vi "NavbalLabVIEW(15-5-28.vi"() -> ()   [LabVIEW 2012] (continued)
            n1742 = Index Array(array=w713, index (col)=0 ("disabled index (col)")) -> (element=w715:string[])  [unwired: 1 in]
            n1743 = for {
              N: w706 -> [_]
              tunnel: w705 -> [w721] mode=indexing
              tunnel: w708 -> [w720] mode=indexing
              tunnel: [w719] -> w709 mode=indexing
              tunnel: w715 -> [w718] mode=indexing
              n1744 = Equal?(x=w718, y="W") -> (x = y?=w716:bool)
              n1745 = case shown="True" w716 {
                tunnel: w721 -> [w727 w735]
                tunnel: w720 -> [w724 w732]
                tunnel: [w722 w730] -> w719
                frame False {
                  n1746 = Decrement(x=w727) -> (x-1=w726:dbl)
                  n1747 = Divide(x=360.0, y=w724) -> (x/y=w723:dbl)
                  n1748 = Multiply(x=w723, y=w726) -> (x*y=w722:dbl)
                }
                frame True {
                  n1749 = Decrement(x=w735) -> (x-1=w734:dbl)
                  n1750 = Divide(x=360.0, y=w732) -> (x/y=w731:dbl)
                  n1751 = Multiply(x=w731, y=w734) -> (x*y=w729:dbl)
                  n1752 = Subtract(x=360.0, y=w729) -> (x-y=w730:dbl)
                }
              }
            }
            n1753 = Reshape Array(w709, 4 ("dimension size"), 1 ("dimension size")) -> (w712:dbl[][])
            n1754 = local write "Correction Phase"(w712) -> ()
          }
          frame #1 {
            w782 = i16 3 ("precision (6)")
            # "Add Correction \nto Baseline Vibes"
            # "Calc Effect of Masses"
            n1755 = local read "Startpt Complex"() -> (w743:cdb[][])
            n1756 = Divide(x="Correction Phase", y=180) -> (x/y=w807:T3)
            n1757 = Complex To Polar(r * e^(i*theta)=w743) -> (r=w795:dbl[][], theta=w796:dbl[][])
            n1758 = call-poly <vilib>:"Multiply.vi"("Real Scalar c"=3.141592653589793, "Real Matrix A"=w807) -> ("A * c"=w805:T3)
            n1759 = Divide(x=w796, y=3.141592653589793) -> (x/y=w792:dbl[][])
            n1760 = local read "Response Coefficients"() -> (w742:cdb[][])
            n1761 = call-poly <vilib>:"Polar To Complex.vi"("Argument Q"=w805, "Modulus r"="Correction Mag") -> ("Complex Matrix r*e^iQ"=w809:T15)
            n1762 = Multiply ("Multiply.vi")(x=w792, y=180) -> (x*y=w797:dbl[][])
            n1763 = call-poly <vilib>:"Matrix To Array.vi"("Real Matrix"=w795) -> ("Real 2D Array"=w770:dbl[][])
            n1764 = call-poly <vilib>:"Array To Matrix.vi"("Complex 2D Array"=w743) -> ("Complex Matrix"=w762:T15)
            n1765 = call-poly <vilib>:"A x B.vi"("B"=w809, "A"=w742) -> ("A x B"=w751:T15)  [unwired: 1 out]
            n1766 = Matrix Size(0:w797) -> (1:w799:i32)  [unwired: 1 out]
            n1767 = Index Array(array=w770, index (col)=0 ("disabled index (col)")) -> (element=w764:dbl[])  [unwired: 1 in]
            n1768 = call-poly <vilib>:"Add.vi"("Complex Matrix B"=w762, "Complex Matrix A"=w751) -> ("A + B"=w771:T15)
            n1769 = Matrix Size(0:w762) -> (1:w791:i32)  [unwired: 1 out]
            n1770 = Square(x=w764) -> (x^2=w768:dbl[])
            n1771 = for {
              N: w799 -> [_]
              tunnel: w797 -> [w813] mode=indexing
              tunnel: [w814] -> w798 mode=indexing
              n1772 = Index Array(array=w813, index=0) -> (element=w811:dbl)
              n1773 = Add(x=360.0, y=w811) -> (x+y=w815:dbl)
              n1774 = Less Than 0?(x=w811) -> (x < 0?=w816:bool)
              n1775 = Select(t=w815, s=w816, f=w811) -> (s? t:f=w814:dbl)
            }
            n1776 = Add Array Elements(numeric array=w768) -> (sum=w767:dbl)
            n1777 = call-poly <vilib>:"Complex To Polar.vi"("Complex Matrix r*e^iQ"=w771) -> ("Modulus r"=w737:T3, "Argument Q"=w757:T3)
            n1778 = Divide(x=w767, y=w791) -> (x/y=w766:dbl)
            n1779 = call-poly <vilib>:"Multiply.vi"("Real Scalar c"=180.0 ("y"), "Real Matrix A"=w757) -> ("A * c"=w759:T3)
            n1780 = Square Root(x=w766) -> (sqrt(x)=w765:dbl)
            n1781 = Divide(x=w759, y=3.141592653589793) -> (x/y=w761:T3)
            n1782 = Absolute Value(x=w765) -> (abs(x)=w778:dbl)
            n1783 = Round To Nearest(number=w761) -> (nearest integer value=w790:T3)
            n1784 = call-poly <vilib>:"Subtract.vi"("Real Matrix B"=w737, "Real Matrix A"=w795) -> ("A - B"=w773:T3)
            n1785 = call-poly <vilib>:"Matrix To Array.vi"("Real Matrix"=w737) -> ("Real 2D Array"=w752:dbl[][])
            n1786 = Matrix Size(0:w790) -> (1:w763:i32)  [unwired: 1 out]
            n1787 = Index Array(array=w752, index (col)=0 ("disabled index (col)")) -> (element=w772:dbl[])  [unwired: 1 in]
            n1788 = for {
              N: w763 -> [_]
              tunnel: w790 -> [w820] mode=indexing
              tunnel: [w821] -> w736 mode=indexing
              n1789 = Index Array(array=w820, index=0) -> (element=w818:dbl)
              n1790 = Add(x=360.0, y=w818) -> (x+y=w822:dbl)
              n1791 = Less Than 0?(x=w818) -> (x < 0?=w823:bool)
              n1792 = Select(t=w822, s=w823, f=w818) -> (s? t:f=w821:dbl)
            }
            "Predicted Phase" <- w736
            n1793 = Build Array (concatenate)(w795, w798, w737, w736, w773) -> (w774:T3)
            n1794 = Array Max & Min(array=w737) -> (max index (indices)=w750:i32[])  [unwired: 3 out]
            n1795 = Square(x=w772) -> (x^2=w754:dbl[])
            n1796 = Add Array Elements(numeric array=w754) -> (sum=w755:dbl)
            n1797 = Index Array(array=w750, index=0) -> (element=w748:i32)
            n1798 = Number To Fractional String(number=w774, precision (6)=w782) -> (F-format string=w775:string[][])  [unwired: 2 in]
            n1799 = Divide(x=w755, y=w791) -> (x/y=w756:dbl)
            n1800 = Number To Fractional String(number=w778, precision (6)=w782) -> (F-format string=w788:string)  [unwired: 2 in]
            n1801 = Square Root(x=w756) -> (sqrt(x)=w777:dbl)
            n1802 = Insert Into Array(array=w775, index (row)=w791, new element=string[] [] ("new element/subarray")) -> (w779:string[][])  [unwired: 1 in]
            n1803 = Bundle(w748, "disabled index (col)"=3) -> (w800:cluster{i32, "disabled index (col)":i32})  [unwired: 1 in]
            n1804 = Concatenate Strings("RMS: " ("string"), w788) -> (w789:string)
            n1805 = Replace Array Subset(array=w779, new element=w789, index (row)=w791, index (col)=0 ("disabled index (col)")) -> (w781:string[][])
            n1806 = property on="Prediction Results" class="MCListbox (strict)"("ActiveCell"=w800) -> (error out=w747:errorcluster)  [unwired: 2 in, 1 out]
            n1807 = Number To Fractional String(number=w777, precision (6)=w782) -> (F-format string=w784:string)  [unwired: 2 in]
            n1808 = Concatenate Strings("RMS: " ("string"), w784) -> (w786:string)
            n1809 = Replace Array Subset(array=w781, new element=w786, index (row)=w791, index (col)=2 ("disabled index (col)")) -> (w746:string[][])
            n1810 = property on="Prediction Results" class="MCListbox (strict)"(error in=w747, "CellBG"=u32 16759409) -> ()  [unwired: 1 in, 2 out]
            n1811 = call-poly <vilib>:"Matrix To Array.vi"("Real Matrix"=w737) -> ("Real 2D Array"=w740:dbl[][])
            n1812 = local read "Sensor Column"() -> (w741:string[])
            n1813 = Index Array(array=w740, index (col)=0 ("disabled index (col)")) -> (element=→"Predicted Mag":dbl[])  [unwired: 1 in]
            n1814 = Insert Into Array(array=w746, index (col)=0 ("disabled index (col)"), new element=w741) -> (w745:string[][])  [unwired: 1 in]
            n1815 = property on="Prediction Results" class="MCListbox (strict)"("ItemNames"=w745) -> ()  [unwired: 2 in, 2 out]
          }
        }
        n1816 = local read "Select Side to Analyze"() -> (w634:enum32{"Starboard", "Port"})
        n1817 = case "True: Structure to create and store new Solutions\n\nFalse:  Structure to Forward Selected Solution to Weight Split and Prediction Tabs" shown="True" "Calculate Solution" {
          tunnel: w603 -> [_ w1831]
          tunnel: w602 -> [_ w1830]
          frame False {
            n1818 = invoke on="Solution Options" class="MCListbox (strict)" method="Get DblClk Row"() -> ("Get Double-clicked Row"=w1689:i32)  [unwired: 3 in, 2 out]
            n1819 = Not Equal?(x=w1689, y=-2.0) -> (x != y?=w1691:bool)
            n1820 = case shown="True" w1691 {
              tunnel: w1689 -> [_ w1714]
              frame False {
                # "no button pressed, \n\ndont do anything stupid."
              }
              frame True {
                w1692 = dbl[][] [[0.0], [0.0], [0.0], [0.0]]
                # "Loops restore trivial planes (previously removed for solving) to data"
                # "when a solution is double-clicked, forward it to the weight Splitter and Prediction inputs"
                n1821 = case shown="0, Default" w1714 {
                  tunnel: [w1801 w1803 w1805 w1807 w1809 w1811 w1813 w1815 w1817 w1819 w1821 w1823 w1825 w1827 w1829] -> w1710
                  tunnel: [w1800 w1802 w1804 w1806 w1808 w1810 w1812 w1814 w1816 w1818 w1820 w1822 w1824 w1826 w1828] -> w1700
                  frame 0, Default {
                    n1822 = local read "Final Phase 0"() -> (w1800:T3)
                    n1823 = local read "Final Mag 0"() -> (w1801:T3)
                  }
                  frame 1 {
                    n1824 = local read "Final Phase 1"() -> (w1802:T3)
                    n1825 = local read "Final Mag 1"() -> (w1803:T3)
                  }
                  frame 2 {
                    n1826 = local read "Final Phase 2"() -> (w1804:T3)
                    n1827 = local read "Final Mag  2"() -> (w1805:T3)
                  }
                  frame 3 {
                    n1828 = local read "Final Phase 3"() -> (w1806:T3)
                    n1829 = local read "Final Mag 3"() -> (w1807:T3)
                  }
                  frame 4 {
                    n1830 = local read "Final Phase 4"() -> (w1808:T3)
                    n1831 = local read "Final Mag 4"() -> (w1809:T3)
                  }
                  frame 5 {
                    n1832 = local read "Final Phase 5"() -> (w1810:T3)
                    n1833 = local read "Final Mag  5"() -> (w1811:T3)
                  }
                  frame 6 {
                    n1834 = local read "Final Phase 6"() -> (w1812:T3)
                    n1835 = local read "Final Mag  6"() -> (w1813:T3)
                  }
                  frame 7 {
                    n1836 = local read "Final Phase 7"() -> (w1814:T3)
                    n1837 = local read "Final Mag  7"() -> (w1815:T3)
                  }
                  frame 8 {
                    n1838 = local read "Final Phase 8"() -> (w1816:T3)
                    n1839 = local read "Final Mag 8"() -> (w1817:T3)
                  }
                  frame 9 {
                    n1840 = local read "Final Phase 9"() -> (w1818:T3)
                    n1841 = local read "Final Mag 9"() -> (w1819:T3)
                  }
                  frame 10 {
                    n1842 = local read "Final Phase 10"() -> (w1820:T3)
                    n1843 = local read "Final Mag 10"() -> (w1821:T3)
                  }
                  frame 11 {
                    n1844 = local read "Final Phase 11"() -> (w1822:T3)
                    n1845 = local read "Final Mag 11"() -> (w1823:T3)
                  }
                  frame 12 {
                    n1846 = local read "Final Phase 12"() -> (w1824:T3)
                    n1847 = local read "Final Mag 12"() -> (w1825:T3)
                  }
                  frame 13 {
                    n1848 = local read "Final Phase 13"() -> (w1826:T3)
                    n1849 = local read "Final Mag 13"() -> (w1827:T3)
                  }
                  frame 14 {
                    n1850 = local read "Final Phase 14"() -> (w1828:T3)
                    n1851 = local read "Final Mag 14"() -> (w1829:T3)
                  }
                }
                n1852 = property on="Solution Options" class="MCListbox (strict)"("SelColor"=u32 40727) -> ()  [unwired: 2 in, 2 out]
                n1853 = Initialize Array(0.0 ("element"), 4 ("dimension size"), 1 ("dimension size")) -> (w1709:dbl[][])
                n1854 = Initialize Array(0.0 ("element"), 4 ("dimension size"), 1 ("dimension size")) -> (w1704:dbl[][])
                n1855 = for {
                  N: 4 -> [_]
                  tunnel: w1710 -> [w1782]
                  shift-right: [w1785] -> w1699
                  shift-left: w1709 -> [w1784]
                  shift-right: [w1778] -> _
                  shift-left: 0 ("dimension size") -> [w1779]
                  i -> [w1783]
                  # "Check if plane was used"
                  n1856 = case shown="0, Default" w1783 {
                    tunnel: [w1796 w1797 w1798 w1799] -> w1786
                    frame 0, Default {
                      n1857 = local read "1st Available"() -> (w1796:bool)
                    }
                    frame 1 {
                      n1858 = local read "2nd Available"() -> (w1797:bool)
                    }
                    frame 2 {
                      n1859 = local read "3rd Available"() -> (w1798:bool)
                    }
                    frame 3 {
                      n1860 = local read "4th Available"() -> (w1799:bool)
                    }
                  }
                  n1861 = Index Array(array=w1782, index (row)=w1779, index (col)=0 ("index (row)")) -> (element=w1781:dbl)
                  n1862 = case shown="True" w1786 {
                    tunnel: w1781 -> [_ w1792]
                    tunnel: [w1788 w1793] -> w1785
                    tunnel: w1783 -> [_ w1794]
                    tunnel: w1784 -> [w1788 w1795]
                    tunnel: w1779 -> [w1787 w1790]
                    tunnel: [w1787 w1789] -> w1778
                    frame False {
                      # "If plane was not used:\nDo nothing\ncheck next plane"
                    }
                    frame True {
                      # "If plane was used:\nadd that data to new matrix\nand then look to next plane"
                      n1863 = Increment(x=w1790) -> (x+1=w1789:i32)
                      n1864 = Replace Array Subset(array=w1795, new element=w1792, index (row)=w1794, index (col)=0 ("disabled index (col)")) -> (w1793:dbl[][])
                    }
                  }
                }
                n1865 = for {
                  N: 4 -> [_]
                  tunnel: w1700 -> [w1760]
                  shift-right: [w1763] -> w1698
                  shift-left: w1704 -> [w1762]
                  shift-right: [w1757] -> _
                  shift-left: 0 ("dimension size") -> [w1758]
                  i -> [w1761]
                  n1866 = case shown="0, Default" w1761 {
                    tunnel: [w1774 w1775 w1776 w1777] -> w1764
                    frame 0, Default {
                      n1867 = local read "1st Available"() -> (w1774:bool)
                    }
                    frame 1 {
                      n1868 = local read "2nd Available"() -> (w1775:bool)
                    }
                    frame 2 {
                      n1869 = local read "3rd Available"() -> (w1776:bool)
                    }
                    frame 3 {
                      n1870 = local read "4th Available"() -> (w1777:bool)
                    }
                  }
                  n1871 = Index Array(array=w1760, index (row)=w1758, index (col)=0 ("index (row)")) -> (element=w1753:dbl)
                  n1872 = Less Than 0?(x=w1753) -> (x < 0?=w1756:bool)
                  n1873 = Add(x=w1753, y=360) -> (x+y=w1754:dbl)
                  n1874 = Select(t=w1754, s=w1756, f=w1753) -> (s? t:f=w1752:dbl)
                  n1875 = case shown="True" w1764 {
                    tunnel: w1752 -> [_ w1770]
                    tunnel: [w1766 w1771] -> w1763
                    tunnel: w1761 -> [_ w1772]
                    tunnel: w1762 -> [w1766 w1773]
                    tunnel: w1758 -> [w1765 w1768]
                    tunnel: [w1765 w1767] -> w1757
                    frame False {
                    }
                    frame True {
                      n1876 = Increment(x=w1768) -> (x+1=w1767:i32)
                      n1877 = Replace Array Subset(array=w1773, new element=w1770, index (row)=w1772, index (col)=0 ("disabled index (col)")) -> (w1771:dbl[][])
                    }
                  }
                }
                n1878 = local read "With/Against\nRotation"() -> (w1694:string[][])
                n1879 = local write "Correction Mag"(w1699) -> ()
                n1880 = local read "Divisions in\nEach Plane"() -> (w1697:T3)
                n1881 = local write "Ideal Weight"(w1699) -> ()
                n1882 = for {
                  tunnel: w1698 -> [w1724] mode=indexing
                  tunnel: [w1723] -> w1695 mode=indexing
                  tunnel: w1697 -> [w1722]
                  tunnel: w1694 -> [w1721]
                  tunnel: [w1718] -> w1693 mode=indexing
                  i -> [w1720]
                  n1883 = Index Array(array=w1721, index (row)=w1720, index (col)=0 ("disabled index (col)")) -> (element=w1717:string)
                  n1884 = Equal?(x=w1717, y="W") -> (x = y?=w1715:bool)
                  n1885 = case shown="True" w1715 {
                    tunnel: w1724 -> [w1725 w1744]
                    tunnel: [w1730 w1740] -> w1723
                    tunnel: w1722 -> [w1729 w1748]
                    tunnel: w1720 -> [w1728 w1747]
                    tunnel: [w1725 w1734] -> w1718
                    frame False {
                      n1886 = Index Array(array=w1729, index (row)=w1728, index (col)=0 ("disabled index (col)")) -> (element=w1727:dbl)
                      n1887 = Divide(x=w1727, y=sgl 360.0) -> (x/y=w1732:dbl)
                      n1888 = Multiply(x=w1725, y=w1732) -> (x*y=w1731:dbl[])
                      n1889 = Increment(x=w1731) -> (x+1=w1730:dbl[])
                    }
                    frame True {
                      w1736 = dbl[] [0.0]
                      w1742 = sgl 360.0 ("y")
                      n1890 = Index Array(array=w1748, index (row)=w1747, index (col)=0 ("disabled index (col)")) -> (element=w1746:dbl)
                      n1891 = Divide(x=w1746, y=sgl 360.0) -> (x/y=w1750:dbl)
                      n1892 = Subtract(x=w1742, y=w1744) -> (x-y=w1735:dbl[])
                      n1893 = Replace Array Subset(array=w1736, new element=w1742, index=0 ("index (row)")) -> (w1741:dbl[])
                      n1894 = Equal?(x=w1735, y=w1741) -> (x = y?=w1739:bool[])
                      n1895 = Index Array(array=w1739, index=0) -> (element=w1737:bool)
                      n1896 = Select(t=w1736, s=w1737, f=w1735) -> (s? t:f=w1734:dbl[])
                      n1897 = Multiply(x=w1734, y=w1750) -> (x*y=w1749:dbl[])
                      n1898 = Increment(x=w1749) -> (x+1=w1740:dbl[])
                    }
                  }
                }
                "Location" <- w1695
                n1899 = property on="wt1" class="Arr (strict)"("Value"=w1692) -> ()  [unwired: 2 in, 2 out]
                n1900 = property on="loc1" class="Arr (strict)"("Value"=w1692) -> ()  [unwired: 2 in, 2 out]
                n1901 = property on="loc2" class="Arr (strict)"("Value"=w1692) -> ()  [unwired: 2 in, 2 out]
                n1902 = property on="wt2" class="Arr (strict)"("Value"=w1692) -> ()  [unwired: 2 in, 2 out]
                n1903 = local write "Degrees"(w1693) -> ()
                n1904 = local write "Correction Loc"(w1695) -> ()
              }
            }
          }
          frame True {
            n1905 = stacked-sequence {
              tunnel: w1831 -> [w1833 _]
              tunnel: w1830 -> [w1832 _]
              frame #0 {
                w1855 = 0.0 ("Final RMS 12")
                w1856 = T3 [[0.0], [0.0], [0.0], [0.0]] ("Initial Mag 5")
                # "Clear List Box in Preparation for New Solutions"
                # "Reset All Previous Solution Results on new solve."
                n1906 = local write "Final Mag 1"(w1856) -> ()
                n1907 = local write "Final Mag  2"(w1856) -> ()
                n1908 = local write "Final Mag 3"(w1856) -> ()
                n1909 = local write "Final Mag 4"(w1856) -> ()
                n1910 = local write "Final Mag  5"(w1856) -> ()
                n1911 = local write "Final Mag 8"(w1856) -> ()
                n1912 = local write "Final Mag  7"(w1856) -> ()
                n1913 = local write "Final Mag  6"(w1856) -> ()
                n1914 = local write "Final Mag 9"(w1856) -> ()
                n1915 = local write "Final Mag 10"(w1856) -> ()
                n1916 = local write "Final Mag 11"(w1856) -> ()
                n1917 = local write "Final Mag 12"(w1856) -> ()
                n1918 = local write "Final Mag 13"(w1856) -> ()
                n1919 = local write "Final Mag 14"(w1856) -> ()
                n1920 = Multiply(x="Start Point:", y=2) -> (x*y=w1848:i32)
                n1921 = local read "DataTab"() -> (w1844:i32)
                n1922 = call <vilib>:"New Report.vi"("report type"=T11."Excel", "template (empty)"=w1832) -> ("report out"=w1838:refnum<class "NI_report.lvclass">, "error out"=w1837:errorcluster)  [unwired: 12 in]
                n1923 = Increment(x=w1848) -> (x+1=w1850:i32)
                n1924 = local write "Final Phase 1"(w1856) -> ()
                n1925 = local write "Final Phase 2"(w1856) -> ()
                n1926 = local write "Final Phase 3"(w1856) -> ()
                n1927 = local write "Final Phase 4"(w1856) -> ()
                n1928 = local write "Final Phase 5"(w1856) -> ()
                n1929 = local write "Final Phase 6"(w1856) -> ()
                n1930 = local write "Final Phase 7"(w1856) -> ()
                n1931 = local write "Final Phase 8"(w1856) -> ()
                n1932 = local write "Final Phase 9"(w1856) -> ()
                n1933 = local write "Final Phase 10"(w1856) -> ()
                n1934 = local write "Final Phase 11"(w1856) -> ()
                n1935 = local write "Final Phase 12"(w1856) -> ()
                n1936 = local write "Final Phase 13"(w1856) -> ()
                n1937 = local write "Final Phase 14"(w1856) -> ()
                n1938 = Bundle("y"=12, w1850) -> (w1841:cluster{"y":i32, i32})  [unwired: 1 in]
                n1939 = call <vilib>:"Excel Get Worksheet.vi"("report in"=w1838, "worksheet index (0)"=w1844, "error in (no error)"=w1837) -> ("report out"=w1835:refnum<class "NI_report.lvclass">, "error out"=w1834:errorcluster)  [unwired: 11 out]
                n1940 = Increment(x=w1850) -> (x+1=w1849:i32)
                n1941 = Bundle(w1833, w1849) -> (w1842:cluster{i32, i32})  [unwired: 1 in]
                n1942 = call-poly <vilib>:"Excel Get Data.vi"("report in"=w1835, "data type"=string[][] [], "start (-1, -1)"=w1841, "end (-1, -1)"=w1842, "error in (no error)"=w1834) -> ("data"=w1843:string[][], "error out"=w1846:errorcluster)  [unwired: 9 out]
                n1943 = local write "Resid 1"(w1855) -> ()
                n1944 = local write "Resid 2"(w1855) -> ()
                n1945 = local write "Resid 3"(w1855) -> ()
                n1946 = local write "Resid 4"(w1855) -> ()
                n1947 = local write "Resid 5"(w1855) -> ()
                n1948 = local write "Resid 6"(w1855) -> ()
                n1949 = local write "Resid 7"(w1855) -> ()
                n1950 = local write "Resid 8"(w1855) -> ()
                n1951 = local write "Resid 9"(w1855) -> ()
                n1952 = local write "Resid 10"(w1855) -> ()
                n1953 = local write "Resid 11"(w1855) -> ()
                n1954 = local write "Resid 12"(w1855) -> ()
                n1955 = local write "Resid 13"(w1855) -> ()
                n1956 = local write "Resid 14"(w1855) -> ()
                n1957 = Fract/Exp String To Number(string=w1843) -> (number=→"Solution Startpoint":dbl[][])  [unwired: 3 in, 1 out]
                n1958 = call <vilib>:"General Error Handler.vi"("error in (no error)"=w1846) -> ()  [unwired: 2 in, 13 out]
                n1959 = Number To Fractional String(number=T3 [[0.0]] ("Initial Mag 5"), precision (6)=i16 3) -> (F-format string=w1852:string[][])  [unwired: 2 in]
                n1960 = property on="Solution Options" class="MCListbox (strict)"("ItemNames"=w1852) -> ()  [unwired: 2 in, 2 out]
              }
              frame #1 {
                w1869 = 180  # Degrees
                # "Response Coeff"
                # "Base"
                # "Find # of Planes\nto solve for"
                # "Input Current Baseline Data"
                # "Do not solve for Planes with no Response Coefficients"
                n1961 = local read "Solution Startpoint"() -> (w1857:sgl[][])
                n1962 = local read "Response Coefficients"() -> (w1870:cdb[][])
                n1963 = for {
                  N: 4 -> [_]
                  shift-right: [w1888] -> w1881
                  shift-left: w1870 -> [w1889]
                  i -> [w1887]
                  n1964 = Subtract(x=3, y=w1887) -> (x-y=w1885:i32)
                  n1965 = case shown="2" w1885 {
                    tunnel: [w1895 w1896 w1897 w1898] -> w1890
                    frame 0, Default {
                      n1966 = local read "1st Available"() -> (w1895:bool)
                    }
                    frame 1 {
                      n1967 = local read "2nd Available"() -> (w1896:bool)
                    }
                    frame 2 {
                      n1968 = local read "3rd Available"() -> (w1897:bool)
                    }
                    frame 3 {
                      n1969 = local read "4th Available"() -> (w1898:bool)
                    }
                  }
                  n1970 = case shown="False" w1890 {
                    tunnel: w1889 -> [w1893 w1894]
                    tunnel: [w1892 w1894] -> w1888
                    tunnel: w1885 -> [w1891 _]
                    frame False {
                      n1971 = Delete From Array(array=w1893, index (col)=w1891) -> (array with subset deleted=w1892:cdb[][])  [unwired: 2 in, 1 out]
                    }
                    frame True {
                    }
                  }
                }
                n1972 = Array Size(array=w1857) -> (size(s)=w1868:i32[])
                n1973 = Index Array(array=w1868, index=1) -> (element=w1861:i32)
                n1974 = Build Array("Solution Weighting Array", "Solution Weighting Array", "Solution Weighting Array", "Solution Weighting Array") -> (w1874:dbl[][])
                n1975 = Transpose 2D Array(2D array=w1874) -> (transposed array=w1873:dbl[][])
                n1976 = Array Subset "Magnitude Column"(array=w1857, index (col)=0 ("index"), length (col)=w1861) -> (w1859:sgl[][])  [unwired: 2 in]
                n1977 = Matrix Size(0:w1881) -> (2:w1884:i32)  [unwired: 1 out]
                n1978 = Array Subset "Phase Column"(array=w1857, index (col)=1 ("index"), length (col)=w1861) -> (w1863:sgl[][])  [unwired: 2 in]
                n1979 = Complex To Polar(r * e^(i*theta)=w1881) -> (r=w1880:dbl[][], theta=w1879:dbl[][])
                n1980 = Divide(x=w1863, y=w1869) -> (x/y=w1864:sgl[][])
                n1981 = Multiply(x=w1873, y=w1859) -> (x*y=w1860:dbl[][])
                n1982 = Multiply(x=w1880, y=w1873) -> (x*y=w1878:dbl[][])
                n1983 = Multiply(x=w1864, y=3.141592653589793) -> (x*y=w1858:dbl[][])
                n1984 = property on="Solution Options" class="MCListbox (strict)"("SelColor"=u32 2771455) -> ()  [unwired: 2 in, 2 out]
                n1985 = Polar To Complex(1:w1858, 2:w1860) -> (0:w1872:cdb[][])
                n1986 = Polar To Complex(1:w1879, 2:w1878) -> (0:w1877:cdb[][])
                n1987 = Polar To Complex(1:w1858, 2:w1859) -> (0:→"Startpt Complex":cdb[][])
                n1988 = call-poly <vilib>:"Array To Matrix.vi"("Complex 2D Array"=w1872) -> ("Complex Matrix"=w1883:T15)
                n1989 = case shown="4" w1884 {
                  tunnel: w1877 -> [w1911 w1953 w2057 w2266]
                  tunnel: w1883 -> [w1910 w1952 w2056 w2265]
                  frame 1, Default {
                    # "Find Which Solution has \nLowest Max residual"
                    # "Store Solution Data\nin Advanced Tab"
                    # "Force Program to Ignore Iterative Solution\n(Navbal Solution)"
                    # "Arrange Data for Listbox"
                    # "One Plane was available:\n\nFind solution using that plane"
                    n1990 = call "SolutionCalculator (SubVI) (2).vi"("Iterative?"="Iterative Solution?", "Max Iteration Count"="Max Iteration Count", "Base Run (matrix)"=w1910, "Response Coefficients"=w1911) -> ("Correction Phase (radians)"=w1903:T3, "RMS Residual"=w1901:dbl, "Correction Mag"=w1907:T3)  [unwired: 1 out]
                    "Resid 0" <- w1901
                    "Final Mag 0" <- w1907
                    n1991 = call-poly <vilib>:"Multiply.vi"("Real Scalar c"=180.0 ("y"), "Real Matrix A"=w1903) -> ("A * c"=w1905:T3)
                    n1992 = Initialize Array(0.0 ("element"), 4 ("dimension size"), 1 ("dimension size")) -> (w1916:dbl[][])
                    n1993 = Divide(x=w1905, y=3.141592653589793) -> (x/y=→"Final Phase 0":T3)
                    n1994 = for "Restore Information to Columns of unused planes" {
                      N: 4 -> [_]
                      tunnel: w1907 -> [w1934]
                      shift-right: [w1937] -> w1914
                      shift-left: w1916 -> [w1936]
                      shift-right: [w1930] -> _
                      shift-left: 0 ("dimension size") -> [w1931]
                      i -> [w1935]
                      n1995 = case shown="3" w1935 {
                        tunnel: [w1948 w1949 w1950 w1951] -> w1938
                        frame 0, Default {
                          n1996 = local read "1st Available"() -> (w1948:bool)
                        }
                        frame 1 {
                          n1997 = local read "2nd Available"() -> (w1949:bool)
                        }
                        frame 2 {
                          n1998 = local read "3rd Available"() -> (w1950:bool)
                        }
                        frame 3 {
                          n1999 = local read "4th Available"() -> (w1951:bool)
                        }
                      }
                      n2000 = Index Array(array=w1934, index (row)=w1931, index (col)=0 ("index (row)")) -> (element=w1933:dbl)
                      n2001 = case shown="True" w1938 {
                        tunnel: w1933 -> [_ w1944]
                        tunnel: [w1940 w1945] -> w1937
                        tunnel: w1935 -> [_ w1946]
                        tunnel: w1936 -> [w1940 w1947]
                        tunnel: w1931 -> [w1939 w1942]
                        tunnel: [w1939 w1941] -> w1930
                        frame False {
                        }
                        frame True {
                          n2002 = Increment(x=w1942) -> (x+1=w1941:i32)
                          n2003 = Replace Array Subset(array=w1947, new element=w1944, index (row)=w1946, index (col)=0 ("disabled index (col)")) -> (w1945:dbl[][])
                        }
                      }
                    }
                    n2004 = Transpose Matrix(1:w1914) -> (0:w1915:dbl[][])
                    n2005 = Build Array (concatenate)(w1915, w1901) -> (w1920:T3)
                    n2006 = Number To Fractional String(number=w1920, precision (6)=i16 3) -> (F-format string=w1900:string[][])  [unwired: 2 in]
                    n2007 = for {
                      tunnel: w1900 -> [w1923] mode=indexing
                      tunnel: [w1922] -> w1899 mode=indexing
                      n2008 = for {
                        tunnel: w1923 -> [w1924] mode=indexing
                        tunnel: [w1925] -> w1922 mode=indexing
                        n2009 = Equal?(x="0.000", y=w1924) -> (x = y?=w1926:bool)
                        n2010 = case shown="False" w1926 {
                          tunnel: [w1928 ""] -> w1925
                          tunnel: w1924 -> [w1928 _]
                          frame False {
                          }
                          frame True {
                          }
                        }
                      }
                    }
                    n2011 = property on="Solution Options" class="MCListbox (strict)"("ItemNames"=w1899) -> ()  [unwired: 2 in, 2 out]
                  }
                  frame 2 {
                    # "2 Planes were available:\n\nRun solver for all combinations of those 2 planes\n\nOrder:\n0) Both Planes\n1) First Plane Only\n2) Last Plane Only"
                    n2012 = for {
                      N: 3 -> [_]
                      tunnel: w1953 -> [w1956]
                      tunnel: w1952 -> [w1955]
                      i -> [w1957]
                      # "Inner Case #2 is Commented"
                      n2013 = case shown="1" w1957 {
                        tunnel: w1956 -> [w1968 w1983 w2022]
                        tunnel: w1955 -> [w1967 w1986 w2006]
                        frame 0, Default {
                          n2014 = local read "Max Iteration Count"() -> (w1966:dbl)
                          n2015 = local read "Iterative Solution?"() -> (w1965:bool)
                          n2016 = call "SolutionCalculator (SubVI) (2).vi"("Iterative?"=w1965, "Max Iteration Count"=w1966, "Base Run (matrix)"=w1967, "Response Coefficients"=w1968) -> ("Correction Phase (radians)"=w1960:T3, "RMS Residual"=w1958:dbl, "Correction Mag"=w1964:T3)  [unwired: 1 out]
                          n2017 = call-poly <vilib>:"Multiply.vi"("Real Scalar c"=180.0 ("y"), "Real Matrix A"=w1960) -> ("A * c"=w1962:T3)
                          n2018 = Divide(x=w1962, y=3.141592653589793) -> (x/y=w1959:T3)
                          n2019 = local write "Resid 0"(w1958) -> ()
                          n2020 = local write "Final Phase 0"(w1959) -> ()
                          n2021 = local write "Final Mag 0"(w1964) -> ()
                        }
                        frame 1 {
                          w1987 = 2  # Plane Number
                          n2022 = Decrement(x=w1987) -> (x-1=w1980:i32)
                          n2023 = Delete From Array(array=w1983, index (col)=w1980) -> (array with subset deleted=w1982:cdb[][])  [unwired: 2 in, 1 out]
                          n2024 = local read "Max Iteration Count"() -> (w1985:dbl)
                          n2025 = local read "Iterative Solution?"() -> (w1984:bool)
                          n2026 = call "SolutionCalculator (SubVI) (2).vi"("Iterative?"=w1984, "Max Iteration Count"=w1985, "Base Run (matrix)"=w1986, "Response Coefficients"=w1982) -> ("Correction Phase (radians)"=w1978:T3, "RMS Residual"=→"Resid 1":dbl, "Correction Mag"=w1979:T3)  [unwired: 1 out]
                          n2027 = call-poly <vilib>:"Polar To Complex.vi"("Argument Q"=w1978, "Modulus r"=w1979) -> ("Complex Matrix r*e^iQ"=w1977:T15)
                          n2028 = Insert Into Array(array=w1977, index (row)=w1980, new element=cdb[] [0.0+0.0i, 0.0+0.0i] ("new element/subarray")) -> (w1976:T15)  [unwired: 1 in]
                          n2029 = call-poly <vilib>:"Complex To Polar.vi"("Complex Matrix r*e^iQ"=w1976) -> ("Modulus r"=→"Final Mag 1":T3, "Argument Q"=w1971:T3)
                          n2030 = call-poly <vilib>:"Multiply.vi"("Real Scalar c"=180.0 ("y"), "Real Matrix A"=w1971) -> ("A * c"=w1973:T3)
                          n2031 = Divide(x=w1973, y=3.141592653589793) -> (x/y=→"Final Phase 1":T3)
                        }
                        frame 2 {
                          w2023 = 1  # Plane Number
                          # "First Plane is restored with Zeros\nsince it was unused in the solution"
                          # "Restore palceholders for plane which were unavailable for use in solution (uncalculated Response Coeffs)"
                          # "Case 2 excludes the\nfirst plane,\n\nso this column is removed\nfrom the response Coeff\nbefore proceding"
                          n2032 = local read "Max Iteration Count"() -> (w2004:dbl)
                          n2033 = local read "Iterative Solution?"() -> (w2003:bool)
                          n2034 = Decrement(x=w2023) -> (x-1=w2001:i32)
                          n2035 = Delete From Array(array=w2022, index (col)=w2001) -> (array with subset deleted=w2005:cdb[][])  [unwired: 2 in, 1 out]
                          n2036 = call "SolutionCalculator (SubVI) (2).vi"("Iterative?"=w2003, "Max Iteration Count"=w2004, "Base Run (matrix)"=w2006, "Response Coefficients"=w2005) -> ("Correction Phase (radians)"=w1991:T3, "RMS Residual"=w1990:dbl, "Correction Mag"=w1992:T3)  [unwired: 1 out]
                          "Resid 2" <- w1990
                          n2037 = call-poly <vilib>:"Polar To Complex.vi"("Argument Q"=w1991, "Modulus r"=w1992) -> ("Complex Matrix r*e^iQ"=w2000:T15)
                          n2038 = Insert Into Array(array=w2000, index (row)=w2001, new element=cdb[] [0.0+0.0i, 0.0+0.0i] ("new element/subarray")) -> (w1999:T15)  [unwired: 1 in]
                          n2039 = call-poly <vilib>:"Complex To Polar.vi"("Complex Matrix r*e^iQ"=w1999) -> ("Modulus r"=w1998:T3, "Argument Q"=w1994:T3)
                          "Final Mag  2" <- w1998
                          n2040 = local read "Final Mag 1"() -> (w2018:T3)
                          n2041 = local read "Final Mag 0"() -> (w2017:T3)
                          n2042 = call-poly <vilib>:"Multiply.vi"("Real Scalar c"=180.0 ("y"), "Real Matrix A"=w1994) -> ("A * c"=w1996:T3)
                          n2043 = Divide(x=w1996, y=3.141592653589793) -> (x/y=→"Final Phase 2":T3)
                          n2044 = Build Array (concatenate)(w2017, w2018, w1998) -> (w2008:T3)
                          n2045 = Initialize Array(0.0 ("element"), 3 ("dimension size"), 2 ("dimension size")) -> (w2011:dbl[][])
                          n2046 = for {
                            N: 4 -> [_]
                            tunnel: w2008 -> [w2039]
                            shift-right: [w2042] -> w2007
                            shift-left: w2011 -> [w2041]
                            shift-right: [w2038] -> _
                            shift-left: 0 ("dimension size") -> [w2034]
                            i -> [w2040]
                            n2047 = case shown="0, Default" w2040 {
                              tunnel: [w2052 w2053 w2054 w2055] -> w2043
                              frame 0, Default {
                                n2048 = local read "1st Available"() -> (w2052:bool)
                              }
                              frame 1 {
                                n2049 = local read "2nd Available"() -> (w2053:bool)
                              }
                              frame 2 {
                                n2050 = local read "3rd Available"() -> (w2054:bool)
                              }
                              frame 3 {
                                n2051 = local read "4th Available"() -> (w2055:bool)
                              }
                            }
                            n2052 = Index Array(array=w2039, index (row)=w2034) -> (element=w2036:dbl[])  [unwired: 1 in]
                            n2053 = Reshape Array(w2036, 1 ("dimension size"), 3 ("dimension size")) -> (w2035:dbl[][])
                            n2054 = Transpose Matrix(1:w2035) -> (0:w2037:dbl[][])
                            n2055 = case shown="True" w2043 {
                              tunnel: w2037 -> [_ w2048]
                              tunnel: [w2045 w2047] -> w2042
                              tunnel: w2040 -> [_ w2046]
                              tunnel: w2041 -> [w2045 w2049]
                              tunnel: w2034 -> [w2044 w2051]
                              tunnel: [w2044 w2050] -> w2038
                              frame False {
                              }
                              frame True {
                                n2056 = Insert Into Array(array=w2049, index (col)=w2046, new element=w2048) -> (w2047:dbl[][])  [unwired: 1 in]
                                n2057 = Increment(x=w2051) -> (x+1=w2050:i32)
                              }
                            }
                          }
                          n2058 = local read "Resid 0"() -> (w2015:dbl)
                          n2059 = local read "Resid 1"() -> (w2016:dbl)
                          n2060 = Build Array(w2015, w2016, w1990) -> (w2019:T3)
                          n2061 = Build Array (concatenate)(w2007, w2019) -> (w2021:T3)
                          n2062 = Number To Fractional String(number=w2021, precision (6)=i16 3) -> (F-format string=w1989:string[][])  [unwired: 2 in]
                          n2063 = for {
                            tunnel: w1989 -> [w2025] mode=indexing
                            tunnel: [w2024] -> w1988 mode=indexing
                            n2064 = for {
                              tunnel: w2025 -> [w2026] mode=indexing
                              tunnel: [w2027] -> w2024 mode=indexing
                              n2065 = Equal?(x="0.000", y=w2026) -> (x = y?=w2028:bool)
                              n2066 = case shown="False" w2028 {
                                tunnel: [w2030 ""] -> w2027
                                tunnel: w2026 -> [w2030 _]
                                frame False {
                                }
                                frame True {
                                }
                              }
                            }
                          }
                          n2067 = property on="Solution Options" class="MCListbox (strict)"("ItemNames"=w1988) -> ()  [unwired: 2 in, 2 out]
                        }
                      }
                    }
                  }
                  frame 3 {
                    # "Refer to 2-Plane Case #2 for commented Inner Structure"
                    # "3 Planes were available:\n\nRun solver for all combinations of those 3 planes\n\nOrder:\n0) 1-1-1\n1) 1-0-1\n2) 0-1-1\n3) 1-1-0\n4) 1-0-0\n5) 0-1-0\n6) 0-0-1"
                    n2068 = for {
                      N: 7 -> [_]
                      tunnel: w2057 -> [w2060]
                      tunnel: w2056 -> [w2059]
                      i -> [w2061]
                      n2069 = case shown="6" w2061 {
                        tunnel: w2060 -> [w2072 w2091 w2111 w2131 w2155 w2179 w2238]
                        tunnel: w2059 -> [w2071 w2079 w2107 w2127 w2145 w2164 w2195]
                        frame 0, Default {
                          n2070 = local read "Max Iteration Count"() -> (w2070:dbl)
                          n2071 = local read "Iterative Solution?"() -> (w2069:bool)
                          n2072 = call "SolutionCalculator (SubVI) (2).vi"("Iterative?"=w2069, "Max Iteration Count"=w2070, "Base Run (matrix)"=w2071, "Response Coefficients"=w2072) -> ("Correction Phase (radians)"=w2064:T3, "RMS Residual"=w2062:dbl, "Correction Mag"=w2068:T3)  [unwired: 1 out]
                          n2073 = local write "Final Mag 0"(w2068) -> ()
                          n2074 = local write "Resid 0"(w2062) -> ()
                          n2075 = call-poly <vilib>:"Multiply.vi"("Real Scalar c"=180.0 ("y"), "Real Matrix A"=w2064) -> ("A * c"=w2066:T3)
                          n2076 = Divide(x=w2066, y=3.141592653589793) -> (x/y=w2063:T3)
                          n2077 = local write "Final Phase 0"(w2063) -> ()
                        }
                        frame 1 {
                          w2092 = 2  # Plane Number
                          n2078 = local read "Max Iteration Count"() -> (w2078:dbl)
                          n2079 = local read "Iterative Solution?"() -> (w2077:bool)
                          n2080 = Decrement(x=w2092) -> (x-1=w2088:i32)
                          n2081 = Delete From Array(array=w2091, index (col)=w2088) -> (array with subset deleted=w2080:cdb[][])  [unwired: 2 in, 1 out]
                          n2082 = call "SolutionCalculator (SubVI) (2).vi"("Iterative?"=w2077, "Max Iteration Count"=w2078, "Base Run (matrix)"=w2079, "Response Coefficients"=w2080) -> ("Correction Phase (radians)"=w2075:T3, "RMS Residual"=w2073:dbl, "Correction Mag"=w2076:T3)  [unwired: 1 out]
                          n2083 = local write "Resid 1"(w2073) -> ()
                          n2084 = call-poly <vilib>:"Polar To Complex.vi"("Argument Q"=w2075, "Modulus r"=w2076) -> ("Complex Matrix r*e^iQ"=w2074:T15)
                          n2085 = Insert Into Array(array=w2074, index (row)=w2088, new element=cdb[] [0.0+0.0i, 0.0+0.0i] ("new element/subarray")) -> (w2089:T15)  [unwired: 1 in]
                          n2086 = call-poly <vilib>:"Complex To Polar.vi"("Complex Matrix r*e^iQ"=w2089) -> ("Modulus r"=w2083:T3, "Argument Q"=w2084:T3)
                          n2087 = call-poly <vilib>:"Multiply.vi"("Real Scalar c"=180.0 ("y"), "Real Matrix A"=w2084) -> ("A * c"=w2086:T3)
                          n2088 = Divide(x=w2086, y=3.141592653589793) -> (x/y=w2082:T3)
                          n2089 = Round To Nearest(number=w2082) -> (nearest integer value=w2081:T3)
                          n2090 = local write "Final Mag 1"(w2083) -> ()
                          n2091 = local write "Final Phase 1"(w2081) -> ()
                        }
                        frame 2 {
                          w2112 = 1  # Plane Number
                          n2092 = local read "Max Iteration Count"() -> (w2106:dbl)
                          n2093 = local read "Iterative Solution?"() -> (w2105:bool)
                          n2094 = Decrement(x=w2112) -> (x-1=w2109:i32)
                          n2095 = Delete From Array(array=w2111, index (col)=w2109) -> (array with subset deleted=w2108:cdb[][])  [unwired: 2 in, 1 out]
                          n2096 = call "SolutionCalculator (SubVI) (2).vi"("Iterative?"=w2105, "Max Iteration Count"=w2106, "Base Run (matrix)"=w2107, "Response Coefficients"=w2108) -> ("Correction Phase (radians)"=w2103:T3, "RMS Residual"=w2093:dbl, "Correction Mag"=w2104:T3)  [unwired: 1 out]
                          n2097 = call-poly <vilib>:"Polar To Complex.vi"("Argument Q"=w2103, "Modulus r"=w2104) -> ("Complex Matrix r*e^iQ"=w2102:T15)
                          n2098 = local write "Resid 2"(w2093) -> ()
                          n2099 = Insert Into Array(array=w2102, index (row)=w2109, new element=cdb[] [0.0+0.0i, 0.0+0.0i] ("new element/subarray")) -> (w2094:T15)  [unwired: 1 in]
                          n2100 = call-poly <vilib>:"Complex To Polar.vi"("Complex Matrix r*e^iQ"=w2094) -> ("Modulus r"=w2100:T3, "Argument Q"=w2096:T3)
                          n2101 = call-poly <vilib>:"Multiply.vi"("Real Scalar c"=180.0 ("y"), "Real Matrix A"=w2096) -> ("A * c"=w2098:T3)
                          n2102 = Divide(x=w2098, y=3.141592653589793) -> (x/y=w2095:T3)
                          n2103 = Round To Nearest(number=w2095) -> (nearest integer value=w2101:T3)
                          n2104 = local write "Final Phase 2"(w2101) -> ()
                          n2105 = local write "Final Mag  2"(w2100) -> ()
                        }
                        frame 3 {
                          w2132 = 3  # Plane Number
                          n2106 = local read "Max Iteration Count"() -> (w2126:dbl)
                          n2107 = local read "Iterative Solution?"() -> (w2125:bool)
                          n2108 = Decrement(x=w2132) -> (x-1=w2129:i32)
                          n2109 = Delete From Array(array=w2131, index (col)=w2129) -> (array with subset deleted=w2128:cdb[][])  [unwired: 2 in, 1 out]
                          n2110 = call "SolutionCalculator (SubVI) (2).vi"("Iterative?"=w2125, "Max Iteration Count"=w2126, "Base Run (matrix)"=w2127, "Response Coefficients"=w2128) -> ("Correction Phase (radians)"=w2123:T3, "RMS Residual"=→"Resid 3":dbl, "Correction Mag"=w2124:T3)  [unwired: 1 out]
                          n2111 = call-poly <vilib>:"Polar To Complex.vi"("Argument Q"=w2123, "Modulus r"=w2124) -> ("Complex Matrix r*e^iQ"=w2122:T15)
                          n2112 = Insert Into Array(array=w2122, index (row)=w2129, new element=cdb[] [0.0+0.0i, 0.0+0.0i] ("new element/subarray")) -> (w2114:T15)  [unwired: 1 in]
                          n2113 = call-poly <vilib>:"Complex To Polar.vi"("Complex Matrix r*e^iQ"=w2114) -> ("Modulus r"=→"Final Mag 3":T3, "Argument Q"=w2116:T3)
                          n2114 = call-poly <vilib>:"Multiply.vi"("Real Scalar c"=180.0 ("y"), "Real Matrix A"=w2116) -> ("A * c"=w2118:T3)
                          n2115 = Divide(x=w2118, y=3.141592653589793) -> (x/y=w2115:T3)
                          n2116 = Round To Nearest(number=w2115) -> (nearest integer value=→"Final Phase 3":T3)
                        }
                        frame 4 {
                          w2151 = 2  # Plane Number
                          w2156 = 3  # Plane Number
                          n2117 = local read "Max Iteration Count"() -> (w2144:dbl)
                          n2118 = local read "Iterative Solution?"() -> (w2143:bool)
                          n2119 = Decrement(x=w2156) -> (x-1=w2153:i32)
                          n2120 = Decrement(x=w2151) -> (x-1=w2150:i32)
                          n2121 = Delete From Array(array=w2155, index (col)=w2153) -> (array with subset deleted=w2152:cdb[][])  [unwired: 2 in, 1 out]
                          n2122 = Delete From Array(array=w2152, index (col)=w2150) -> (array with subset deleted=w2146:cdb[][])  [unwired: 2 in, 1 out]
                          n2123 = call "SolutionCalculator (SubVI) (2).vi"("Iterative?"=w2143, "Max Iteration Count"=w2144, "Base Run (matrix)"=w2145, "Response Coefficients"=w2146) -> ("Correction Phase (radians)"=w2147:T3, "RMS Residual"=→"Resid 4":dbl, "Correction Mag"=w2148:T3)  [unwired: 1 out]
                          n2124 = call-poly <vilib>:"Polar To Complex.vi"("Argument Q"=w2147, "Modulus r"=w2148) -> ("Complex Matrix r*e^iQ"=w2142:T15)
                          n2125 = Insert Into Array(array=w2142, index (row)=1 ("y"), new element=cdb[][] [[0.0+0.0i, 0.0+0.0i], [0.0+0.0i, 0.0+0.0i]] ("new element/subarray")) -> (w2134:T15)  [unwired: 1 in]
                          n2126 = call-poly <vilib>:"Complex To Polar.vi"("Complex Matrix r*e^iQ"=w2134) -> ("Modulus r"=→"Final Mag 4":T3, "Argument Q"=w2136:T3)
                          n2127 = call-poly <vilib>:"Multiply.vi"("Real Scalar c"=180.0 ("y"), "Real Matrix A"=w2136) -> ("A * c"=w2138:T3)
                          n2128 = Divide(x=w2138, y=3.141592653589793) -> (x/y=w2135:T3)
                          n2129 = Round To Nearest(number=w2135) -> (nearest integer value=→"Final Phase 4":T3)
                        }
                        frame 5 {
                          w2173 = T15 [[0.0+0.0i]] ("array")
                          w2176 = 1  # Plane Number
                          w2180 = 3  # Plane Number
                          n2130 = local read "Max Iteration Count"() -> (w2162:dbl)
                          n2131 = local read "Iterative Solution?"() -> (w2161:bool)
                          n2132 = Decrement(x=w2180) -> (x-1=w2178:i32)
                          n2133 = Decrement(x=w2176) -> (x-1=w2175:i32)
                          n2134 = Delete From Array(array=w2179, index (col)=w2178) -> (array with subset deleted=w2177:cdb[][])  [unwired: 2 in, 1 out]
                          n2135 = Delete From Array(array=w2177, index (col)=w2175) -> (array with subset deleted=w2163:cdb[][])  [unwired: 2 in, 1 out]
                          n2136 = call "SolutionCalculator (SubVI) (2).vi"("Iterative?"=w2161, "Max Iteration Count"=w2162, "Base Run (matrix)"=w2164, "Response Coefficients"=w2163) -> ("Correction Phase (radians)"=w2159:T3, "RMS Residual"=→"Resid 5":dbl, "Correction Mag"=w2160:T3)  [unwired: 1 out]
                          n2137 = call-poly <vilib>:"Polar To Complex.vi"("Argument Q"=w2159, "Modulus r"=w2160) -> ("Complex Matrix r*e^iQ"=w2158:T15)
                          n2138 = Build Array (concatenate)(w2173, w2158, w2173) -> (w2174:T15)
                          n2139 = Transpose 2D Array(2D array=w2174) -> (transposed array=w2165:T15)
                          n2140 = call-poly <vilib>:"Complex To Polar.vi"("Complex Matrix r*e^iQ"=w2165) -> ("Modulus r"=→"Final Mag  5":T3, "Argument Q"=w2167:T3)
                          n2141 = call-poly <vilib>:"Multiply.vi"("Real Scalar c"=180.0 ("y"), "Real Matrix A"=w2167) -> ("A * c"=w2169:T3)
                          n2142 = Divide(x=w2169, y=3.141592653589793) -> (x/y=w2166:T3)
                          n2143 = Round To Nearest(number=w2166) -> (nearest integer value=→"Final Phase 5":T3)
                        }
                        frame 6 {
                          w2200 = 0.0 ("element")
                          w2232 = T15 [[0.0+0.0i]] ("array")
                          w2235 = 1  # Plane Number
                          w2239 = 2  # Plane Number
                          # "If plane not available, put zero array"
                          n2144 = local read "Max Iteration Count"() -> (w2194:dbl)
                          n2145 = local read "Iterative Solution?"() -> (w2193:bool)
                          n2146 = Decrement(x=w2239) -> (x-1=w2237:i32)
                          n2147 = Decrement(x=w2235) -> (x-1=w2234:i32)
                          n2148 = Delete From Array(array=w2238, index (col)=w2237) -> (array with subset deleted=w2236:cdb[][])  [unwired: 2 in, 1 out]
                          n2149 = Delete From Array(array=w2236, index (col)=w2234) -> (array with subset deleted=w2196:cdb[][])  [unwired: 2 in, 1 out]
                          n2150 = call "SolutionCalculator (SubVI) (2).vi"("Iterative?"=w2193, "Max Iteration Count"=w2194, "Base Run (matrix)"=w2195, "Response Coefficients"=w2196) -> ("Correction Phase (radians)"=w2197:T3, "RMS Residual"=w2183:dbl, "Correction Mag"=w2198:T3)  [unwired: 1 out]
                          "Resid 6" <- w2183
                          n2151 = call-poly <vilib>:"Polar To Complex.vi"("Argument Q"=w2197, "Modulus r"=w2198) -> ("Complex Matrix r*e^iQ"=w2192:T15)
                          n2152 = local read "3rd Available"() -> (w2212:bool)
                          n2153 = local read "Final Mag 0"() -> (w2228:T3)
                          n2154 = local read "Final Mag 1"() -> (w2229:T3)
                          n2155 = local read "Final Mag  2"() -> (w2224:T3)
                          n2156 = local read "Final Mag 3"() -> (w2223:T3)
                          n2157 = local read "Final Mag 4"() -> (w2222:T3)
                          n2158 = local read "Final Mag  5"() -> (w2221:T3)
                          n2159 = local read "2nd Available"() -> (w2213:bool)
                          n2160 = local read "4th Available"() -> (w2211:bool)
                          n2161 = local read "1st Available"() -> (w2214:bool)
                          n2162 = Build Array (concatenate)(w2232, w2232, w2192) -> (w2233:T15)
                          n2163 = Transpose 2D Array(2D array=w2233) -> (transposed array=w2185:T15)
                          n2164 = Build Array(w2214, w2213, w2212, w2211) -> (w2210:bool[])
                          n2165 = call-poly <vilib>:"Complex To Polar.vi"("Complex Matrix r*e^iQ"=w2185) -> ("Modulus r"=w2216:T3, "Argument Q"=w2187:T3)
                          "Final Mag  6" <- w2216
                          n2166 = Build Array (concatenate)(w2228, w2229, w2224, w2223, w2222, w2221, w2216) -> (w2204:T3)
                          n2167 = Array Size(array=w2204) -> (size(s)=w2209:i32[])
                          n2168 = call-poly <vilib>:"Matrix To Array.vi"("Real Matrix"=w2204) -> ("Real 2D Array"=w2203:dbl[][])
                          n2169 = call-poly <vilib>:"Multiply.vi"("Real Scalar c"=180.0 ("y"), "Real Matrix A"=w2187) -> ("A * c"=w2189:T3)
                          n2170 = Initialize Array "Zeros Array"(w2200, w2200, w2200) -> (w2199:dbl[][])
                          n2171 = Divide(x=w2189, y=3.141592653589793) -> (x/y=w2186:T3)
                          n2172 = Index Array(array=w2209, index=1) -> (element=w2202:i32)
                          n2173 = Initialize Array(0.0 ("element"), w2202) -> (w2206:dbl[])
                          n2174 = local read "Resid 0"() -> (w2226:dbl)
                          n2175 = local read "Resid 1"() -> (w2227:dbl)
                          n2176 = local read "Resid 2"() -> (w2220:dbl)
                          n2177 = local read "Resid 3"() -> (w2219:dbl)
                          n2178 = local read "Resid 4"() -> (w2218:dbl)
                          n2179 = local read "Resid 5"() -> (w2217:dbl)
                          n2180 = Round To Nearest(number=w2186) -> (nearest integer value=→"Final Phase 6":T3)
                          n2181 = for {
                            N: 4 -> [_]
                            tunnel: w2210 -> [w2254] mode=indexing
                            tunnel: w2203 -> [w2255]
                            shift-right: [w2252] -> w2201
                            shift-left: w2199 -> [w2251]
                            tunnel: w2206 -> [w2250]
                            shift-right: [w2248] -> _
                            shift-left: 0 -> [w2249]
                            n2182 = Index Array(array=w2255, index (row)=w2249) -> (element=w2253:dbl[])  [unwired: 1 in]
                            n2183 = case shown="True" w2254 {
                              tunnel: w2253 -> [_ w2264]
                              tunnel: [w2258 w2263] -> w2252
                              tunnel: w2251 -> [w2259 w2262]
                              tunnel: w2250 -> [w2257 _]
                              tunnel: w2249 -> [w2256 w2261]
                              tunnel: [w2256 w2260] -> w2248
                              frame False {
                                n2184 = Build Array (concatenate)(w2259, w2257) -> (w2258:dbl[][])
                              }
                              frame True {
                                n2185 = Build Array (concatenate)(w2262, w2264) -> (w2263:dbl[][])
                                n2186 = Increment(x=w2261) -> (x+1=w2260:i32)
                              }
                            }
                          }
                          n2187 = Build Array(w2226, w2227, w2220, w2219, w2218, w2217, w2183) -> (w2225:T3)
                          n2188 = Transpose 2D Array(2D array=w2201) -> (transposed array=w2205:dbl[][])
                          n2189 = Build Array (concatenate)(w2205, w2225) -> (w2231:T3)
                          n2190 = Number To Fractional String(number=w2231, precision (6)=i16 3) -> (F-format string=w2182:string[][])  [unwired: 2 in]
                          n2191 = for {
                            tunnel: w2182 -> [w2241] mode=indexing
                            tunnel: [w2240] -> w2181 mode=indexing
                            n2192 = for {
                              tunnel: w2241 -> [w2242] mode=indexing
                              tunnel: [w2243] -> w2240 mode=indexing
                              n2193 = Equal?(x="0.000", y=w2242) -> (x = y?=w2244:bool)
                              n2194 = case shown="False" w2244 {
                                tunnel: [w2246 ""] -> w2243
                                tunnel: w2242 -> [w2246 _]
                                frame False {
                                }
                                frame True {
                                }
                              }
                            }
                          }
                          n2195 = property on="Solution Options" class="MCListbox (strict)"("ItemNames"=w2181) -> ()  [unwired: 2 in, 2 out]
                        }
                      }
                    }
                  }
                  frame 4 {
                    # "Refer to 2-Plane Case #2 for commented Inner Structure"
                    # "7) 1-1-1-0\n8) 0-1-1-0\n9) 1-0-1-0\n10) 1-1-0-0\n11) 1-0-0-0\n12) 0-1-0-0\n13) 0-0-1-0\n14) 0-0-0-1\n\n1: Plane Used\n0: Plane Excluded"
